vi "12 Simulated DAQmx Signal (x64-2018).vi"(10 "rate":dbl=6000.0, 11 "number of samples":i32=240) -> (0 "error out":errorcluster, 2 "task out":refnum<k21>)   [LabVIEW 2017]
uses:
  <vilib>/DAQmx/configure/timing.llb/DAQmx Timing (Sample Clock).vi
  <vilib>/DAQmx/configure/trigger.llb/DAQmx Trigger.vi
  <vilib>/DAQmx/configure/trigger.llb/DAQmx Start Trigger (Digital Edge).vi
panel:
  out "Waveform Chart":dynamicdata(graph)
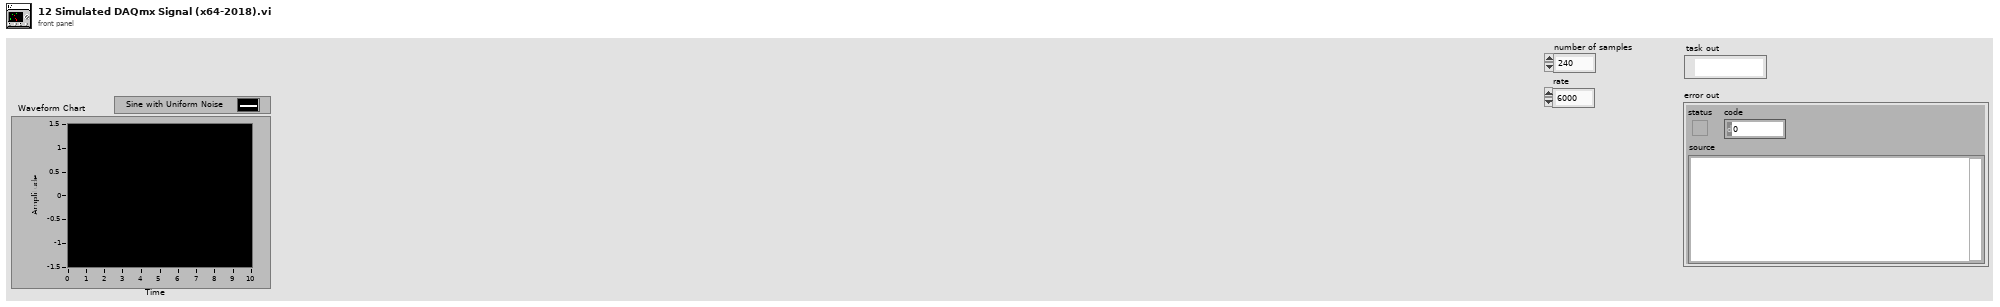
[diagram p1: front panel]
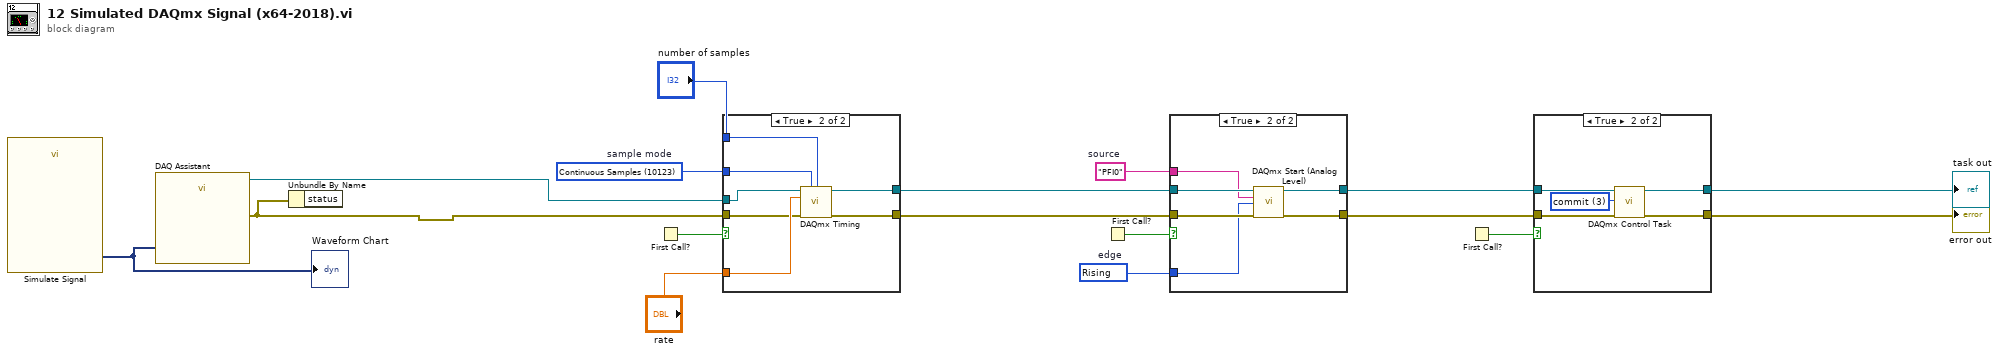
[diagram p0: block diagram]
diagram:
  w13 = 10280 items=["Rising"=10280, "Falling"=10171]  # edge
  w12 = "PFI0"  # source
  w8 = 10123 items=["Finite Samples"=10178, "Continuous Samples"=10123, "Hardware Timed Single Point"=12522]  # sample mode
  n1 = call "Simulate Signal"() -> ("Sine with Uniform Noise"=w3:dynamicdata)  [unwired: 14 in, 1 out]
  "Waveform Chart" <- w3
  n2 = call "DAQ Assistant"("data"=w3) -> ("task out"=w2:refnum<k21>, "error out"=w1:errorcluster)  [unwired: 16 in, 1 out]
  n3 = Unbundle By Name(w1) -> ()  [unwired: 1 out]
  n4 = First Call?() -> (First Call?: T/F=w4:bool)
  n5 = case shown="True" w4 {
    tunnel: [w19 w23] -> w10
    tunnel: [w18 w22] -> w5
    tunnel: "number of samples" -> [_ w26]
    tunnel: w8 -> [_ w25]
    tunnel: "rate" -> [_ w24]
    tunnel: w2 -> [w19 w21]
    tunnel: w1 -> [w18 w20]
    frame False {
    }
    frame True {
      n6 = call-poly <vilib>:"DAQmx Timing.vi"("task/channels in"=w21, "sample mode"=w25, "samples per channel"=w26, "rate"=w24, "error in"=w20) -> ("task out"=w23:refnum<k21>, "error out"=w22:errorcluster)  [unwired: 9 in]
    }
  }
  n7 = First Call?() -> (First Call?: T/F=w9:bool)
  n8 = case shown="True" w9 {
    tunnel: [w28 w32] -> w15
    tunnel: w10 -> [w28 w34]
    tunnel: [w27 w31] -> w11
    tunnel: w5 -> [w27 w33]
    tunnel: w12 -> [_ w30]
    tunnel: w13 -> [_ w29]
    frame False {
    }
    frame True {
      n9 = call-poly "DAQmx Start (Analog Level).vi"("task/channels in"=w34, "source"=w30, "edge"=w29, "error in"=w33) -> ("task out"=w32:refnum<k21>, "error out"=w31:errorcluster)  [unwired: 10 in]
    }
  }
  n10 = First Call?() -> (First Call?: T/F=w14:bool)
  n11 = case shown="True" w14 {
    tunnel: [w36 w40] -> w17
    tunnel: w15 -> [w36 w41]
    tunnel: [w35 w38] -> w16
    tunnel: w11 -> [w35 w39]
    frame False {
    }
    frame True {
      w37 = 3 items=["verify"=2, "reserve"=4, "commit"=3, "unreserve"=5, "abort"=6] ("action")
      n12 = call <vilib>:"DAQmx Control Task.vi"("task/channels in"=w41, "action"=w37, "error in"=w39) -> ("task out"=w40:refnum<k21>, "error out"=w38:errorcluster)  [unwired: 11 in]
    }
  }
  "task out" <- w17
  "error out" <- w16
